vi "Save_Before-After_Tracks-4.vi"(4 "Save movies?":bool, 5 "[IN] Number of event":i8=2, 6 "[IN] Localization Settings":T5 {"[IN] Image Type" items=["Grayscale (U8)", "Grayscale (I16)", "Grayscale (SGL)", "Complex (CSG)", "RGB (U32)", "HSL (U32)", "RGB (U64)", "Grayscale (U16)"]; "[IN] Particle Filter Setups"."Type of particle filter"."Measurement Parameter" items=["Center of Mass X", "Center of Mass Y", "First Pixel X", "First Pixel Y", "Bounding Rect Left", "Bounding Rect Top", "Bounding Rect Right", "Bounding Rect Bottom", "Max Feret Diameter Start X", "Max Feret Diameter Start Y", "Max Feret Diameter End X", "Max Feret Diameter End Y", "Max Horiz. Segment Length Left", "Max Horiz. Segment Length Right", "Max Horiz. Segment Length Row", "-", "Bounding Rect Width", "Bounding Rect Height", "Bounding Rect Diagonal", "Perimeter", "Convex Hull Perimeter", "Holes' Perimeter", "Max Feret Diameter", "Equivalent Ellipse Major Axis", "Equivalent Ellipse Minor Axis", "Equivalent Ellipse Minor Axis (Feret)", "Equivalent Rect Long Side", "Equivalent Rect Short Side", "Equivalent Rect Diagonal", "Equivalent Rect Short Side (Feret)", "Average Horiz. Segment Length", "Average Vert. Segment Length", "Hydraulic Radius", "Waddel Disk Diameter", "-", "Area", "Holes' Area", "Particle & Holes' Area", "Convex Hull Area", "Image Area", "-", "Number of Holes", "Number of Horiz. Segments", "Number of Vert. Segments", "-", "Orientation", "Max Feret Diameter Orientation", "-", "% Area/Image Area", "% Area/(Particle & Holes' Area)", "Ratio of Equivalent Ellipse Axes", "Ratio of Equivalent Rect Sides", "-", "Elongation Factor", "Compactness Factor", "Heywood Circularity Factor", "Type Factor", "-", "Sum X", "Sum Y", "Sum XX", "Sum XY", "Sum YY", "Sum XXX", "Sum XXY", "Sum XYY", "Sum YYY", "-", "Moment of Inertia XX", "Moment of Inertia XY", "Moment of Inertia YY", "Moment of Inertia XXX", "Moment of Inertia XXY", "Moment of Inertia XYY", "Moment of Inertia YYY", "Norm. Moment of Inertia XX", "Norm. Moment of Inertia XY", "Norm. Moment of Inertia YY", "Norm. Moment of Inertia XXX", "Norm. Moment of Inertia XXY", "Norm. Moment of Inertia XYY", "Norm. Moment of Inertia YYY", "Hu Moment 1", "Hu Moment 2", "Hu Moment 3", "Hu Moment 4", "Hu Moment 5", "Hu Moment 6", "Hu Moment 7"]}, 7 "[IN] Images Array":T1[](array[typedef]), 8 "error IN":errorcluster, 9 "[IN] FPS":u32, 10 "default name":string, 11 "[IN] Grouped Tracks Values":T6) -> (0 "error OUT":errorcluster)   [LabVIEW 2013]
doc: "Creation of the *avi file with recorded grouped tracks or tracks with resolved problemss"
uses:
  <vilib>/vision/Avi.llb/IMAQ AVI2 Refnum.ctl
  <vilib>/vision/Image Controls.llb/IMAQ Image.ctl
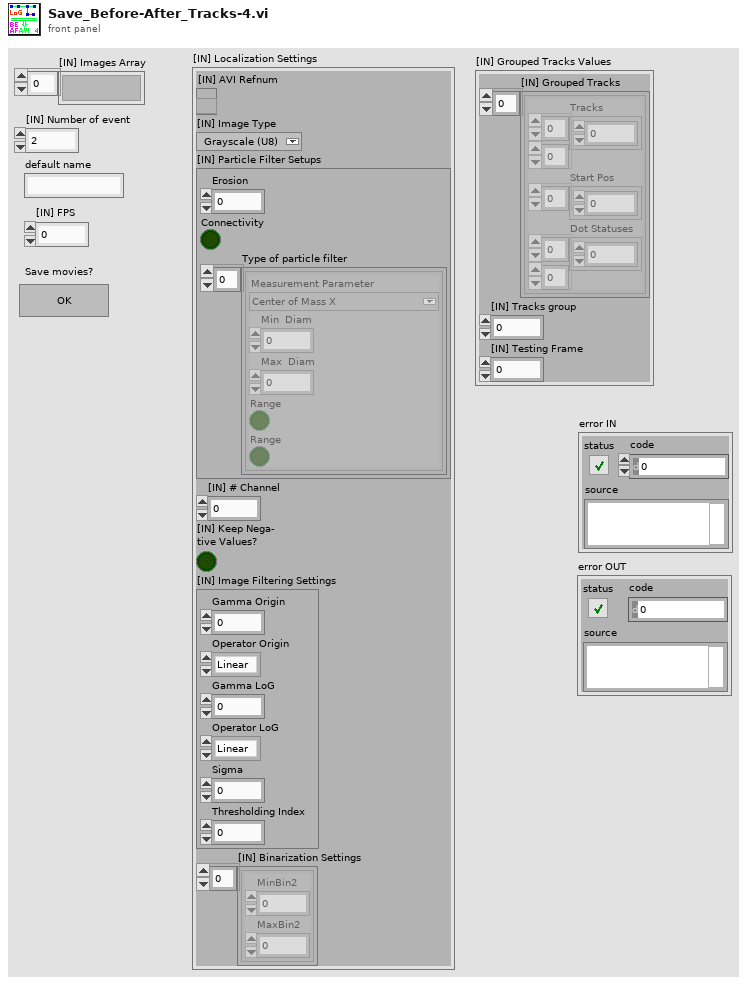
[diagram p1: front panel]
types:
  T1 = typedef "IMAQ Image.ctl" = refnum<image>
  T2 = typedef "IMAQ AVI2 Refnum.ctl" = refnum<k20>
  T3 = typedef "Image Type" = u32
  T4 = typedef "Particle Parameters" = i32
  T5 = cluster{"[IN] AVI Refnum":T2, "[IN] Image Type":T3, "[IN] Particle Filter Setups":cluster{"Erosion":i32, "Connectivity ":bool, "Type of particle filter":cluster{"Measurement Parameter":T4, "Min  Diam":dbl, "Max  Diam":dbl, "Range":bool, "Range":bool}[]}, "[IN] # Channel":u8, "[IN] Keep Nega-\ntive Values?":bool, "[IN] Image Filtering Settings":cluster{"Gamma Origin":sgl, "Operator Origin":enum32{"Linear", "Log", "Exp", "Square", "Square root", "Power X", "Power 1/X"}, "Gamma LoG":sgl, "Operator LoG":enum32{"Linear", "Log", "Exp", "Square", "Square root", "Power X", "Power 1/X"}, "Sigma":dbl, "Thresholding Index":i8}, "[IN] Binarization Settings":cluster{"MinBin2":sgl, "MaxBin2":sgl}[]}
  T6 = cluster{"[IN] Grouped Tracks":cluster{"Tracks":dbl[][], "Start Pos":i32[], "Dot Statuses":i16[][]}[], "[IN] Tracks group":i32, "[IN] Testing Frame ":u32}
  T7 = cluster{"Tracks":dbl[][], "Start Pos":i32[], "Dot Statuses":i16[][]}[]
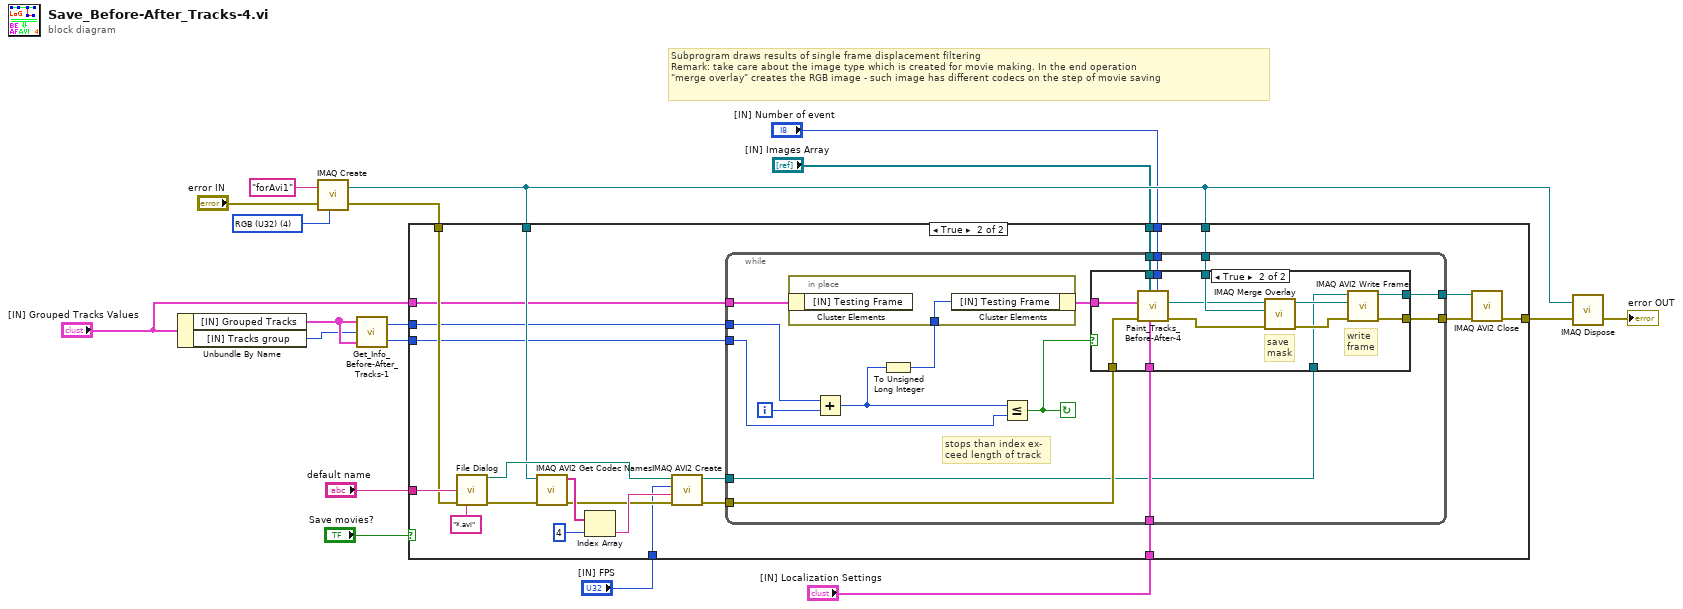
[diagram p0: block diagram]
diagram:
  w12 = T3 4 items=["Grayscale (U8)", "Grayscale (I16)", "Grayscale (SGL)", "Complex (CSG)", "RGB (U32)", "HSL (U32)", "RGB (U64)", "Grayscale (U16)"] ("Image Type")
  # "Subprogram draws results of single frame displacement filtering\nRemark: take care about the image type which is created for movie making. In the end operation\n\"merge overlay\" creates the RGB image - such image has different codecs on the step of movie saving"
  n1 = Unbundle By Name("[IN] Grouped Tracks Values") -> ("[IN] Grouped Tracks"=w6:T7, "[IN] Tracks group"=w5:i32)
  n2 = call "IMAQ Create"("Image Name"="forAvi1", "Image Type"=w12, "error in (no error)"="error IN") -> ("New Image"=w9:T1, "error out"=w8:errorcluster)  [unwired: 2 in]
  n3 = call "Get_Info_Before-After_Tracks-1.vi"("[IN] After Tracks"=w6, "[IN] Tracks group"=w5, "[IN] Before Tracks"=w6) -> ("[OUT] Maximal Frame\n(finish point all tracks)"=w10:i32, "[OUT] Min Start Pos"=w11:i32)
  n4 = case shown="True" "Save movies?" {
    tunnel: w9 -> [_ w27]
    tunnel: "[IN] FPS" -> [_ w35]
    tunnel: [w19 w31] -> w13
    tunnel: "default name" -> [_ w33]
    tunnel: w8 -> [w19 w29]
    tunnel: w11 -> [_ w26]
    tunnel: w10 -> [_ w25]
    tunnel: w9 -> [_ w24]
    tunnel: "[IN] Grouped Tracks Values" -> [_ w23]
    tunnel: "[IN] Localization Settings" -> [_ w22]
    tunnel: "[IN] Images Array" -> [_ w21]
    tunnel: "[IN] Number of event" -> [_ w20]
    frame False {
    }
    frame True {
      n5 = call "File Dialog"("default name"=w33, "error in"=w29, "pattern (all files)"="*.avi") -> ("selected path"=w36:path, "error out"=w34:errorcluster)  [unwired: 9 in, 2 out]
      n6 = call "IMAQ AVI2 Get Codec Names"("error in (no error)"=w34, "Image"=w27) -> ("error out"=w40:errorcluster, "Codec Names"=w42:string[])  [unwired: 8 in]
      n7 = Index Array(array=w42, index=4) -> (element=w41:string)
      n8 = call "IMAQ AVI2 Create"("error in (no error)"=w40, "Codec"=w41, "Frames Per Second"=w35, "AVI Path"=w36) -> ("error out"=w39:errorcluster, "AVI Refnum"=w38:T2)  [unwired: 6 in]
      n9 = while {
        tunnel: w39 -> [w53]
        tunnel: w38 -> [w51]
        tunnel: [w57] -> w32
        tunnel: [w58] -> w30
        tunnel: w26 -> [w55]
        tunnel: w25 -> [w56]
        tunnel: w24 -> [w54]
        tunnel: w23 -> [w48]
        tunnel: w22 -> [w52]
        tunnel: w21 -> [w50]
        tunnel: w20 -> [w49]
        i -> [w46]
        stop <- w43 continue-if-true
        # "stops than index ex-\nceed length of track"
        n10 = Add(x=w55, y=w46) -> (x+y=w44:i32)
        n11 = To Unsigned Long Integer(number=w44) -> (unsigned 32bit integer=w45:u32)
        n12 = in-place {
          in-place-border: w45 -> [w74]
          n13 = in-place-cluster #1(w48) -> ()  [unwired: 1 out]
          n14 = in-place-cluster #1("[IN] Testing Frame"=w74) -> (w47:T6)
        }
        n15 = Less Or Equal?(x=w44, y=w56) -> (x <= y?=w43:bool)
        n16 = case shown="True" w43 {
          tunnel: [w60 w73] -> w58
          tunnel: [w59 w72] -> w57
          tunnel: w54 -> [_ w69]
          tunnel: w53 -> [w59 w68]
          tunnel: w52 -> [_ w67]
          tunnel: w51 -> [w60 w64]
          tunnel: w50 -> [_ w63]
          tunnel: w49 -> [_ w62]
          tunnel: w47 -> [_ w61]
          frame False {
          }
          frame True {
            # "write\nframe"
            # "save\nmask"
            n17 = call "Paint_Tracks_Before-After-4.vi"("[IN] Number of event"=w62, "[IN] Localization Settings"=w67, "[IN] Images Array"=w63, "error IN"=w68, "[IN] Grouped Tracks Values"=w61) -> ("error OUT"=w65:errorcluster, "[OUT] Image with\nDisplacements"=w66:T1)  [unwired: 5 in]
            n18 = call "IMAQ Merge Overlay"("error in (no error)"=w65, "Image Dst"=w69, "Image Src"=w66) -> ("error out"=w70:errorcluster, "Image Dst Out"=w71:T1)  [unwired: 7 in]
            n19 = call "IMAQ AVI2 Write Frame"("error in (no error)"=w70, "Image"=w71, "AVI Refnum"=w64) -> ("error out"=w72:errorcluster, "AVI Refnum (duplicate)"=w73:T2)  [unwired: 6 in, 1 out]
          }
        }
      }
      n20 = call "IMAQ AVI2 Close"("error in (no error)"=w32, "AVI Refnum"=w30) -> ("error out"=w31:errorcluster)  [unwired: 9 in]
    }
  }
  n21 = call "IMAQ Dispose"("Image"=w9, "error in (no error)"=w13) -> ("error out"=→"error OUT":errorcluster)  [unwired: 4 in]
